vi "Framework Configured Test.vi"() -> ()   [LabVIEW 2017]
uses:
  DSF Configuration API/Public/Controls/DSF Engine Framework Configuration.ctl
  DSF Configuration API/Public/Controls/DSF Engine Plugin Configuration.ctl
  DSF Configuration API/Public/Controls/DSF Timing Info.ctl
  DSF Configuration API/Public/Controls/DSF Engine Transfer Group Configuration.ctl
  DSF Configuration API/Public/Controls/DSF Direction.ctl
  DSF Configuration API/Public/Controls/DSF Engine Transfer Configuration.ctl
  DSF Configuration API/Public/Controls/DSF Byte Order.ctl
  DSF Configuration API/Public/Controls/DSF Engine Channel Configuration.ctl
  DSF Configuration API/Public/Controls/DSF Data Type.ctl
  DSF Configuration API/Public/Controls/DSF Settings Info.ctl
  Classes/Framework/Framework Options.ctl
  Typedefs/FIFO Flags.ctl
  Classes/Thread/Thread Options.ctl
  Typedefs/Plugin Flags.ctl
  <vilib>/NI/Memory Manager/Classes/Pointer/Pointer.lvclass
  <vilib>/NI/Memory Manager/Classes/Pointer/Pointer.lvclass/Pointer.ctl
  Classes/Framework/Framework.lvclass
  DSF Core.lvlib
  Classes/Thread/Thread.lvclass
panel:
  out "error out":errorcluster
  in  "initialization options":T1={"FIFO Options"={"Infinite Timeouts"=FALSE}, "Thread Options"={"Show FP On Call"=TRUE, "Close FP After Call"=TRUE}, "Plugin Options"={"Default Components"=TRUE}}
  in  "framework configuration":T5={"components directory"=path "C:/Builds/Data Sharing Framework/Windows/32/Transceivers", "Plugins"=[{"name"="UDP", "class"="UDP", "cycle timing"={"priority"=1000, "decimation"=1, "offset"=0}, "Transfer Groups"=[{"name"="Group0", "direction"=enum."Tx", "cycle timing"={"priority"=100, "decimation"=1, "offset"=0}, "Transfers"=[{"name"="Transfer0", "byte order"=enum."big-endian", "channels"=[{"src buffer offset"=0, "name"="Channel0", "data type"=enum."DBL", "count"=10, "dst buffer offset"=0}], "settings"=[]}], "settings"=[]}], "thread count"=4, "buffer converter settings"=[], "transceiver settings"=[]}, {"name"="GE Reflective Memory", "class"="GE Reflective Memory", "cycle timing"={"priority"=5000, "decimation"=1, "offset"=0}, "Transfer Groups"=[{"name"="Group0", "direction"=enum."Tx", "cycle timing"={"priority"=100, "decimation"=1, "offset"=0}, "Transfers"=[{"name"="Transfer0", "byte order"=enum."big-endian", "channels"=[{"src buffer offset"=0, "name"="Channel0", "data type"=enum."DBL", "count"=10, "dst buffer offset"=0}], "settings"=[]}], "settings"=[]}], "thread count"=1, "buffer converter settings"=[], "transceiver settings"=[]}, {"name"="PXImc", "class"="PXImc", "cycle timing"={"priority"=10000, "decimation"=1, "offset"=0}, "Transfer Groups"=[{"name"="Group0", "direction"=enum."Tx", "cycle timing"={"priority"=100, "decimation"=1, "offset"=0}, "Transfers"=[{"name"="Transfer0", "byte order"=enum."big-endian", "channels"=[{"src buffer offset"=0, "name"="Channel0", "data type"=enum."DBL", "count"=1, "dst buffer offset"=0}], "settings"=[]}], "settings"=[]}], "thread count"=8, "buffer converter settings"=[], "transceiver settings"=[]}]}
  in  "stop":bool
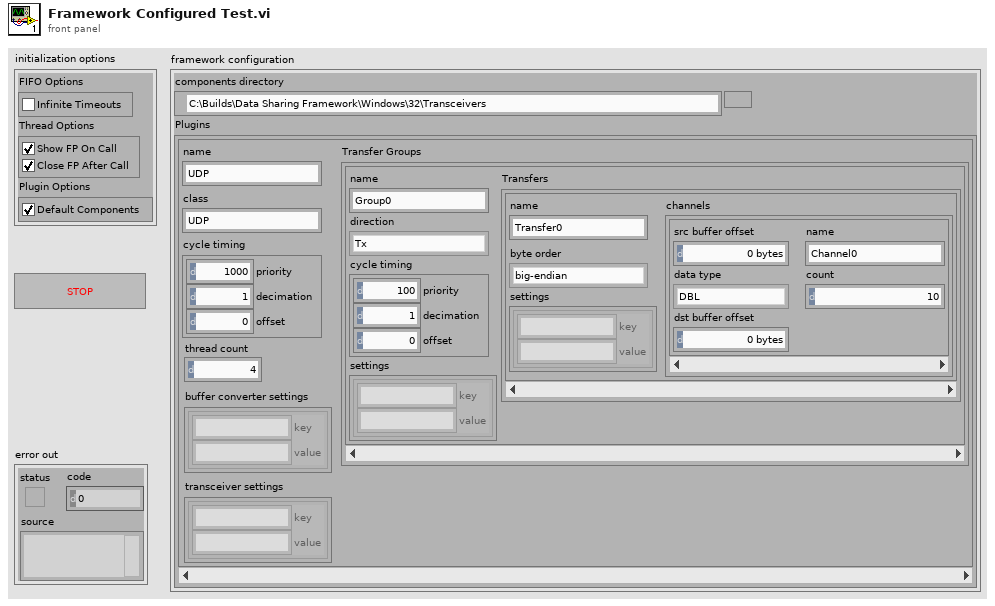
[diagram p1: front panel]
types:
  T1 = typedef "DSF Core.lvlib/Framework.lvclass/Framework Options.ctl" = cluster{"FIFO Options":T2, "Thread Options":T3, "Plugin Options":T4}
  T2 = typedef "DSF Core.lvlib/FIFO Flags.ctl" = cluster{"Infinite Timeouts":bool}
  T3 = typedef "DSF Core.lvlib/Thread.lvclass/Thread Options.ctl" = cluster{"Show FP On Call":bool, "Close FP After Call":bool}
  T4 = typedef "DSF Core.lvlib/Plugin Flags.ctl" = cluster{"Default Components":bool}
  T5 = typedef "DSF Core.lvlib/DSF Engine Framework Configuration.ctl" = cluster{"components directory":path, "Plugins":T6[]}
  T6 = typedef "DSF Core.lvlib/DSF Engine Plugin Configuration.ctl" = cluster{"name":string, "class":string, "cycle timing":T7, "Transfer Groups":T8[], "thread count":i32, "buffer converter settings":T14, "transceiver settings":T14}
  T7 = typedef "DSF Core.lvlib/DSF Timing Info.ctl" = cluster{"priority":u64, "decimation":u64, "offset":u64}
  T8 = typedef "DSF Core.lvlib/DSF Engine Transfer Group Configuration.ctl" = cluster{"name":string, "direction":T9, "cycle timing":T7, "Transfers":T10[], "settings":T14}
  T9 = typedef "DSF Core.lvlib/DSF Direction.ctl" = enum8{"Tx", "Rx"}
  T10 = typedef "DSF Core.lvlib/DSF Engine Transfer Configuration.ctl" = cluster{"name":string, "byte order":T11, "channels":T12[], "settings":T14}
  T11 = typedef "DSF Core.lvlib/DSF Byte Order.ctl" = enum8{"big-endian", "little-endian"}
  T12 = typedef "DSF Core.lvlib/DSF Engine Channel Configuration.ctl" = cluster{"src buffer offset":u64, "name":string, "data type":T13, "count":u64, "dst buffer offset":u64}
  T13 = typedef "DSF Core.lvlib/DSF Data Type.ctl" = enum8{"Bool", "SGL", "DBL", "I8", "I16", "I32", "I64", "U8", "U16", "U32", "U64"}
  T14 = typedef "DSF Core.lvlib/DSF Settings Info.ctl" = cluster{"key":string, "value":string}[]
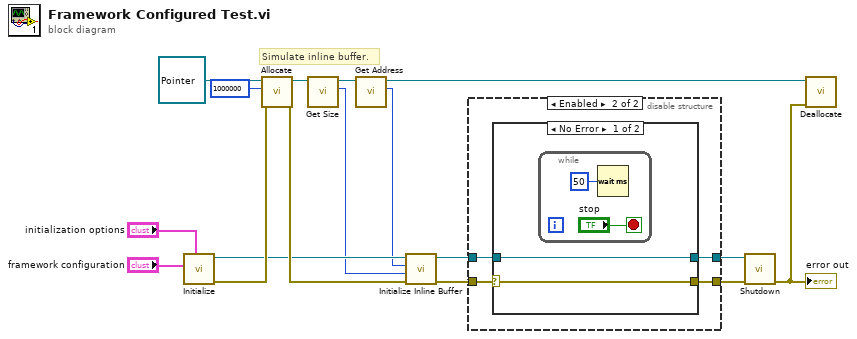
[diagram p0: block diagram]
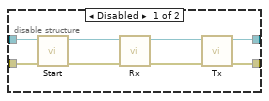
[diagram p2: hidden frame]
diagram:
  # "Simulate inline buffer."
  n1 = call "Initialize.vi"("options"="initialization options", "framework configuration"="framework configuration") -> ("error out"=w8:errorcluster, "Framework out"=w6:refnum<class "Framework.lvclass">)  [unwired: 8 in]
  n2 = call-dynamic "Allocate.vi"("error in (no error)"=w8, "size"=u64 1000000, "Pointer in"=refnum<class "Pointer.lvclass"> refnum) -> ("error out"=w7:errorcluster, "Pointer out"=w10:refnum<class "Pointer.lvclass">)  [unwired: 7 in]
  n3 = call <vilib>:"Get Size.vi"("Pointer in"=w10) -> ("size"=w5:u64, "Pointer out"=w9:refnum<class "Pointer.lvclass">)  [unwired: 9 in]
  n4 = call <vilib>:"Get Address.vi"("Pointer in"=w9) -> ("address"=w4:u64, "Pointer out"=w3:refnum<class "Pointer.lvclass">)  [unwired: 9 in]
  n5 = call "Initialize Inline Buffer.vi"("error in (no error)"=w7, "size"=w5, "address"=w4, "Framework in"=w6) -> ("error out"=w12:errorcluster, "Framework out"=w13:refnum<class "Framework.lvclass">)  [unwired: 6 in]
  n6 = disable-structure shown="Enabled" {
    disable-tunnel: w13 -> [w25 w27]
    disable-tunnel: w12 -> [w24 w29]
    disable-tunnel: [w19 w28] -> w16
    disable-tunnel: [w18 w26] -> w15
    frame Disabled {
      n7 = call "Start.vi"("error in (no error)"=w24, "Framework in"=w25) -> ("error out"=w22:errorcluster, "Framework out"=w23:refnum<class "Framework.lvclass">)  [unwired: 8 in]
      n8 = call "Rx.vi"("error in (no error)"=w22, "Framework in"=w23) -> ("error out"=w20:errorcluster, "Framework out"=w21:refnum<class "Framework.lvclass">)  [unwired: 8 in]
      n9 = call "Tx.vi"("error in (no error)"=w20, "Framework in"=w21) -> ("error out"=w19:errorcluster, "Framework out"=w18:refnum<class "Framework.lvclass">)  [unwired: 8 in]
    }
    frame Enabled {
      n10 = case shown="No Error" w29 {
        selector: w29 -> [w31 w34]
        tunnel: [w31 w34] -> w28
        tunnel: w27 -> [w30 w35]
        tunnel: [w30 w35] -> w26
        frame No Error {
          n11 = while {
            stop <- "stop" stop-if-true
            n12 = Wait (ms)(milliseconds to wait=u32 50) -> ()  [unwired: 1 out]
          }
        }
        frame Error {
        }
      }
    }
  }
  n13 = call "Shutdown.vi"("error in (no error)"=w16, "Framework in"=w15) -> ("error out"=w2:errorcluster)  [unwired: 8 in, 1 out]
  "error out" <- w2
  n14 = call-dynamic "Deallocate.vi"("error in (no error)"=w2, "Pointer in"=w3) -> ()  [unwired: 8 in, 2 out]
